vi "Main.vi"() -> ()   [LabVIEW 2025]
uses:
  Resources/States.ctl
  e90cf40e-0b05-4561-bc81-dadeb3f04810.vi
  <vilib>/Utility/file.llb/Write Delimited Spreadsheet (string).vi
  <vilib>/Comparison/Equal/Equal Functor/Equal Functor.lvclass
panel:
  in  "Back PIN":bool
  in  "Change PIN":bool
  in  "New PIN":i32
  in  "Back":bool
  in  "Withdraw":bool
  in  "Withdrawal Amount":dbl
  in  "Log Out":bool
  in  "Withdrawal":bool
  in  "PIN Change":bool
  in  "Balance":bool
  in  "Exit":bool
  in  "Log In":bool
  in  "PIN":i32
  in  "Card Number":i32
  # "ATM MACHINE"
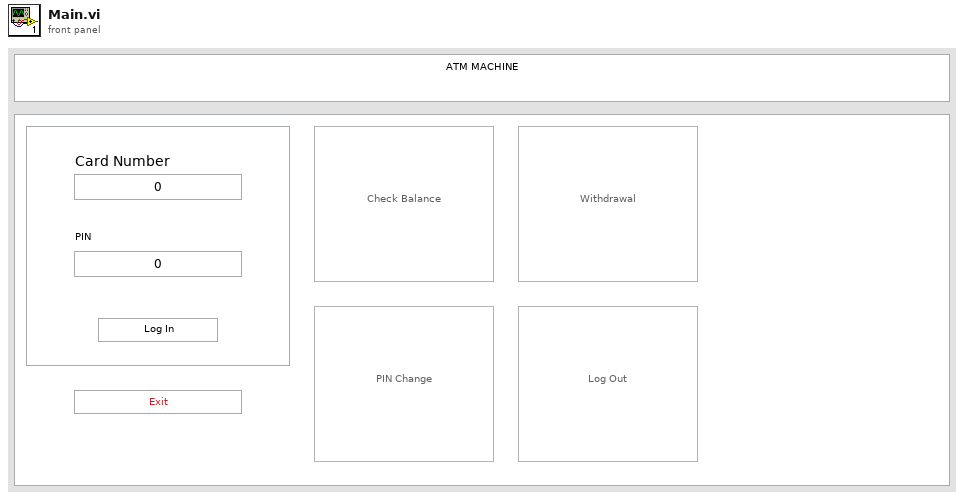
[diagram p1: front panel]
types:
  T1 = cluster{"Card":i32[], "PIN":i32[], "Balance":dbl[], "User Index":i32[]}
  T2 = typedef "States.ctl" = enum16{"Start", "Wait for event", "Log In", "Check Balance", "Withdrawal", "PIN Change", "Money Withdrawal", "Back", "Save File", "New PIN", "Exit Program", "Log Out"}
  T3 = enum16{"open", "replace", "create", "open or create", "replace or create", "replace or create with confirmation"}
  T4 = enum8{"Enabled", "Disabled", "Disabled and Grayed Out"}
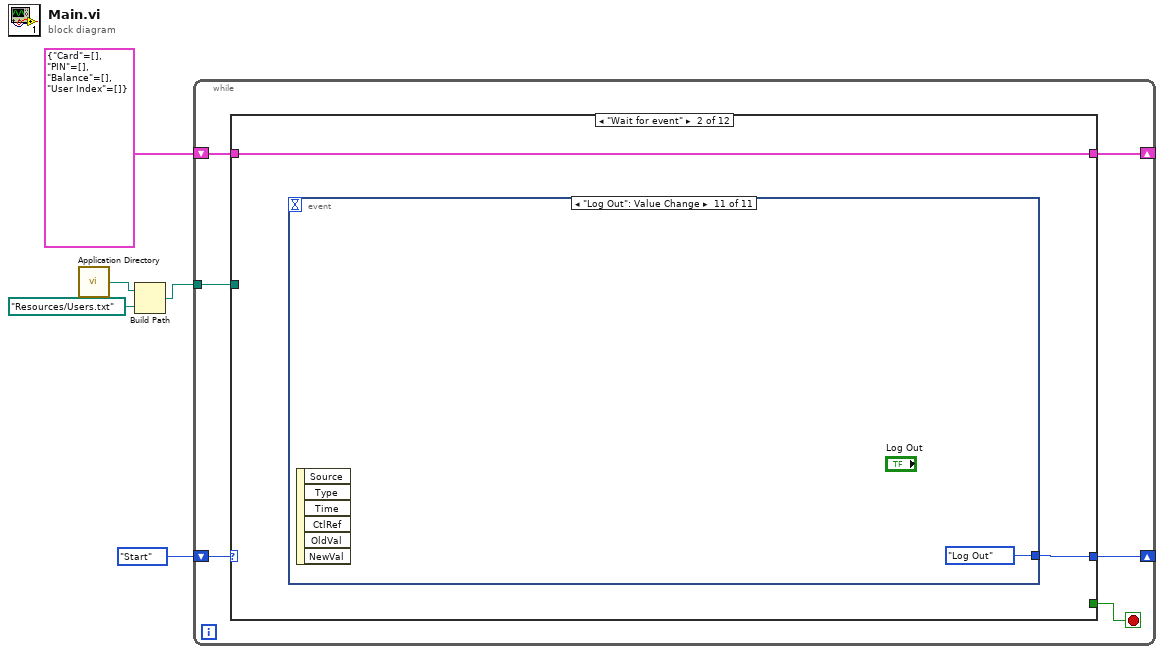
[diagram p0: block diagram]
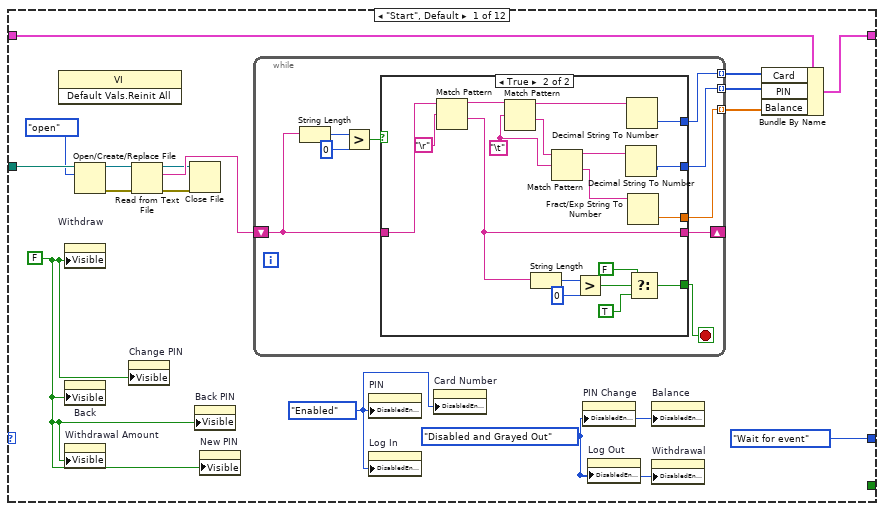
[diagram p2: hidden frame]
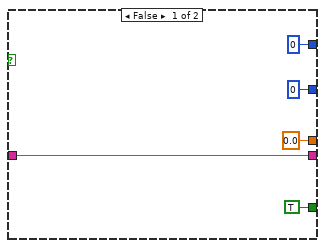
[diagram p3: hidden frame]
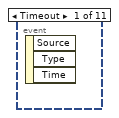
[diagram p4: hidden frame]
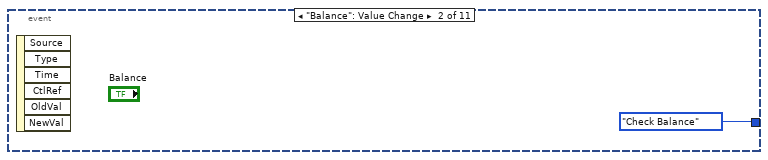
[diagram p5: hidden frame]
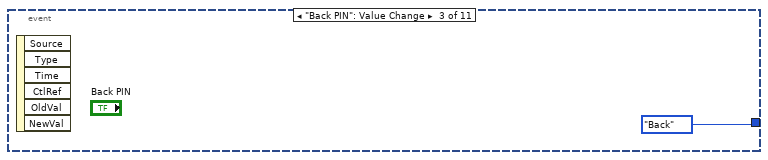
[diagram p6: hidden frame]
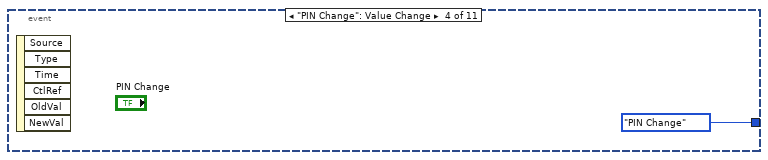
[diagram p7: hidden frame]
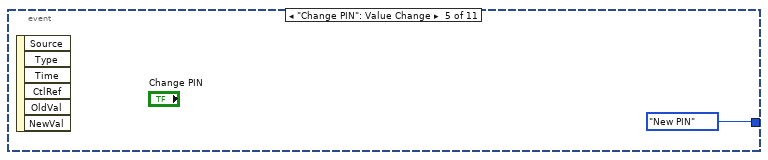
[diagram p8: hidden frame]
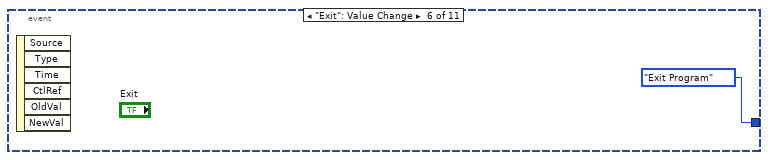
[diagram p9: hidden frame]
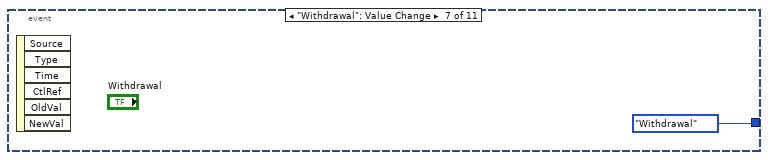
[diagram p10: hidden frame]
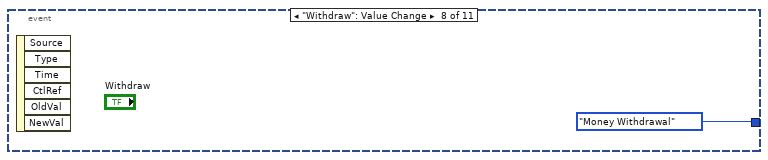
[diagram p11: hidden frame]
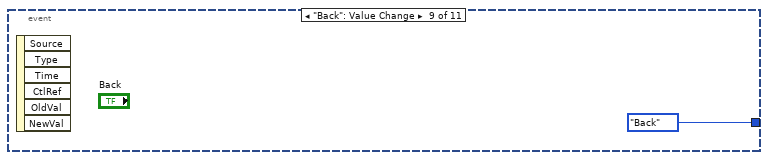
[diagram p12: hidden frame]
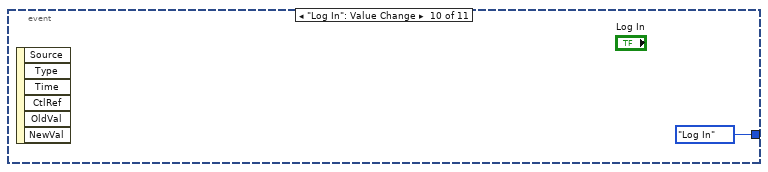
[diagram p13: hidden frame]
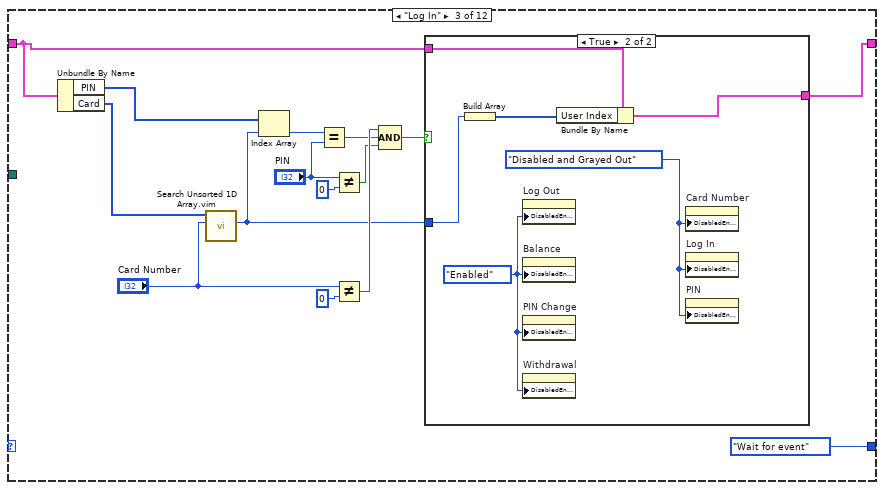
[diagram p14: hidden frame]
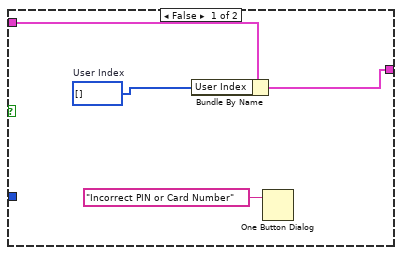
[diagram p15: hidden frame]
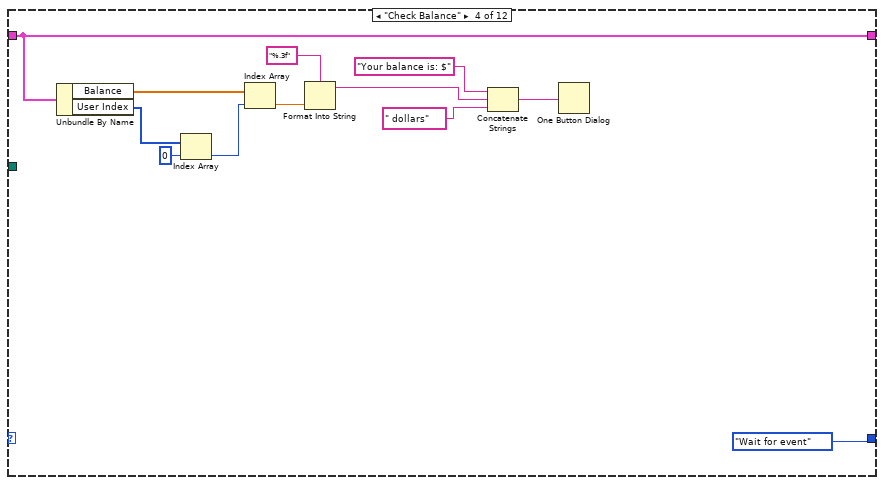
[diagram p16: hidden frame]
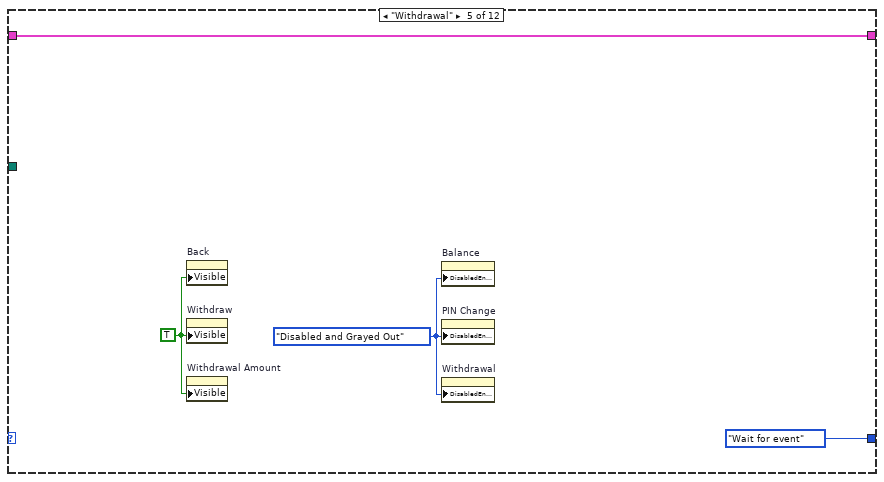
[diagram p17: hidden frame]
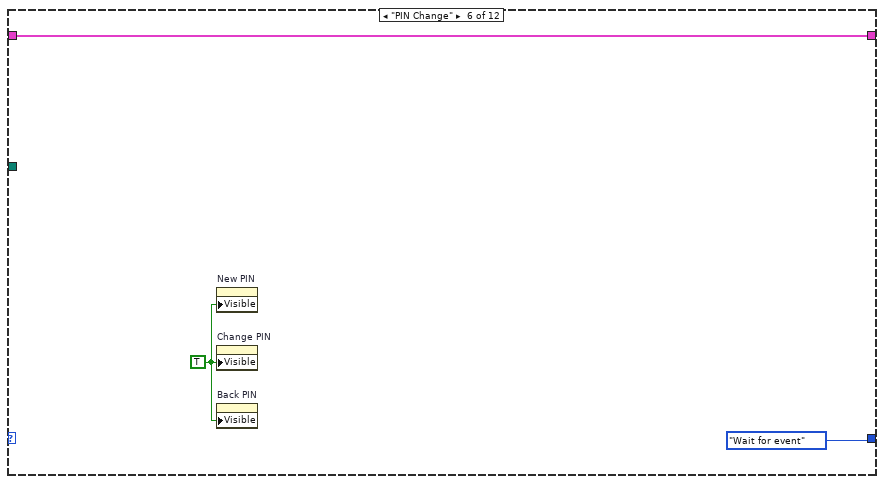
[diagram p18: hidden frame]
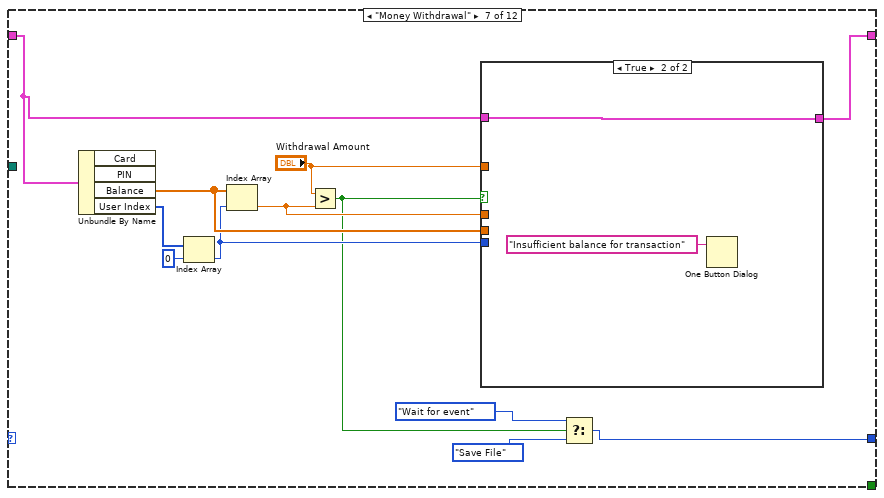
[diagram p19: hidden frame]
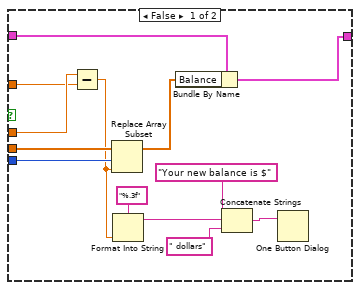
[diagram p20: hidden frame]
diagram:
  n1 = call <vilib>:"Application Directory.vi"() -> ("Application Directory"=w3:path)
  n2 = Build Path(base path=w3, name or relative path=path "Resources/Users.txt") -> (appended path=w1:path)
  n3 = while {
    shift-right: [w10] -> _
    shift-left: States."Start" -> [w11]
    shift-right: [w7] -> _
    shift-left: T1 {"Card"=[], "PIN"=[], "Balance"=[], "User Index"=[]} -> [w8]
    tunnel: w1 -> [w6]
    stop <- w9 stop-if-true
    n4 = case shown="\"Wait for event\"" w11 {
      tunnel: [States."Wait for event" w61 States."Wait for event" States."Wait for event" States."Wait for event" States."Wait for event" w116 States."Wait for event" States."Back" w165 States."Exit Program" States."Start"] -> w10
      tunnel: [_ _ _ _ _ _ _ _ _ _ TRUE _] -> w9
      tunnel: w8 -> [w23 w60 w74 w97 w112 w113 w124 w145 w157 w170 _ _]
      tunnel: [w22 w60 w73 w97 w112 w113 w125 w145 _ w169 _ _] -> w7
      tunnel: w6 -> [w21 _ _ _ _ _ _ _ w148 _ _ _]
      frame "Start", Default {
        w24 = FALSE ("Visible")
        w25 = T4."Disabled and Grayed Out" ("Disabled")
        w26 = T4."Enabled" ("Disabled")
        n5 = invoke class="VI" method="Default Vals.Reinit All"() -> ()  [unwired: 3 in, 3 out]
        n6 = property on="Withdraw" class="Bool"("Visible"=w24) -> ()  [unwired: 2 in, 2 out]
        n7 = property on="Back" class="Bool"("Visible"=w24) -> ()  [unwired: 2 in, 2 out]
        n8 = property on="Withdrawal Amount" class="DigNum (strict)"("Visible"=w24) -> ()  [unwired: 2 in, 2 out]
        n9 = Open/Create/Replace File(file path (use dialog)=w21, operation (0:open)=T3."open") -> (refnum out=w18:refnum<file>, error out=w19:errorcluster)  [unwired: 4 in, 1 out]
        n10 = property on="Change PIN" class="Bool"("Visible"=w24) -> ()  [unwired: 2 in, 2 out]
        n11 = Read from Text File(file (use dialog)=w18, error in=w19) -> (refnum out=w15:refnum<file>, text=w17:string, error out=w16:errorcluster)  [unwired: 2 in, 1 out]
        n12 = Close File(refnum=w15, error in=w16) -> ()  [unwired: 2 out]
        n13 = property on="Back PIN" class="Bool"("Visible"=w24) -> ()  [unwired: 2 in, 2 out]
        n14 = property on="New PIN" class="DigNum (strict)"("Visible"=w24) -> ()  [unwired: 2 in, 2 out]
        n15 = while {
          shift-right: [w36] -> _
          shift-left: w17 -> [w32]
          tunnel: [w30] -> w14 mode=indexing
          tunnel: [w29] -> w13 mode=indexing
          tunnel: [w28] -> w12 mode=indexing
          stop <- w31 stop-if-true
          n16 = String Length(string=w32) -> (length=w35:i32)
          n17 = Greater?(x=w35, y=0) -> (0:w33:bool)
          n18 = case shown="True" w33 {
            tunnel: w32 -> [w41 w59]
            tunnel: [w41 w50] -> w36
            tunnel: [TRUE ("t") w47] -> w31
            tunnel: [0 w45] -> w30
            tunnel: [0 w44] -> w29
            tunnel: [0.0 w43] -> w28
            frame False {
            }
            frame True {
              w42 = "\t"
              n19 = Match Pattern(string=w59, regular expression="\r") -> (before substring=w58:string, after substring=w50:string)  [unwired: 1 in, 2 out]
              n20 = Match Pattern(string=w58, regular expression=w42) -> (before substring=w56:string, after substring=w57:string)  [unwired: 1 in, 2 out]
              n21 = String Length(string=w50) -> (length=w51:i32)
              n22 = Match Pattern(string=w57, regular expression=w42) -> (before substring=w55:string, after substring=w54:string)  [unwired: 1 in, 2 out]
              n23 = Greater?(x=w51, y=0) -> (0:w49:bool)
              n24 = Decimal String To Number(string=w55) -> (number=w44:i32)  [unwired: 2 in, 1 out]
              n25 = Decimal String To Number(string=w56) -> (number=w45:i32)  [unwired: 2 in, 1 out]
              n26 = Fract/Exp String To Number(string=w54) -> (number=w43:dbl)  [unwired: 3 in, 1 out]
              n27 = Select(t=FALSE, s=w49, f=TRUE) -> (s? t:f=w47:bool)
            }
          }
        }
        n28 = property on="PIN" class="DigNum (strict)"("DisabledEnum"=w26) -> ()  [unwired: 2 in, 2 out]
        n29 = property on="Log In" class="Bool"("DisabledEnum"=w26) -> ()  [unwired: 2 in, 2 out]
        n30 = property on="Card Number" class="DigNum (strict)"("DisabledEnum"=w26) -> ()  [unwired: 2 in, 2 out]
        n31 = property on="PIN Change" class="Bool"("DisabledEnum"=w25) -> ()  [unwired: 2 in, 2 out]
        n32 = property on="Log Out" class="Bool"("DisabledEnum"=w25) -> ()  [unwired: 2 in, 2 out]
        n33 = property on="Balance" class="Bool"("DisabledEnum"=w25) -> ()  [unwired: 2 in, 2 out]
        n34 = property on="Withdrawal" class="Bool"("DisabledEnum"=w25) -> ()  [unwired: 2 in, 2 out]
        n35 = Bundle By Name(cluster=w23, "Card"=w14, "PIN"=w13, "Balance"=w12) -> (w22:T1)
      }
      frame "Wait for event" {
        n36 = event shown="[10] \"Log Out\": Value Change" {
          selector: _ -> [_ _ _ _ _ _ _ _ _ _ _]
          dyn-events: _ -> [_ _ _ _ _ _ _ _ _ _ _]
          timeout: _ -> [_ _ _ _ _ _ _ _ _ _ _]
          tunnel: [_ States."Check Balance" States."Back" States."PIN Change" States."New PIN" States."Exit Program" States."Withdrawal" States."Money Withdrawal" States."Back" States."Log In" States."Log Out"] -> w61
          event Timeout {
            n37 = event-data() -> ()  [unwired: 1 in, 3 out]
          }
          event "Balance": Value Change {
            n38 = event-data() -> ()  [unwired: 1 in, 6 out]
          }
          event "Back PIN": Value Change {
            n39 = event-data() -> ()  [unwired: 1 in, 6 out]
          }
          event "PIN Change": Value Change {
            n40 = event-data() -> ()  [unwired: 1 in, 6 out]
          }
          event "Change PIN": Value Change {
            n41 = event-data() -> ()  [unwired: 1 in, 6 out]
          }
          event "Exit": Value Change {
            n42 = event-data() -> ()  [unwired: 1 in, 6 out]
          }
          event "Withdrawal": Value Change {
            n43 = event-data() -> ()  [unwired: 1 in, 6 out]
          }
          event "Withdraw": Value Change {
            n44 = event-data() -> ()  [unwired: 1 in, 6 out]
          }
          event "Back": Value Change {
            n45 = event-data() -> ()  [unwired: 1 in, 6 out]
          }
          event "Log In": Value Change {
            n46 = event-data() -> ()  [unwired: 1 in, 6 out]
          }
          event "Log Out": Value Change {
            n47 = event-data() -> ()  [unwired: 1 in, 6 out]
          }
        }
      }
      frame "Log In" {
        n48 = Unbundle By Name(w74) -> ("PIN"=w76:i32[], "Card"=w75:i32[])
        n49 = call "Search Unsorted 1D Array.vim"("element"="Card Number", "unsorted 1D array"=w75) -> ("index of element"=w72:i32)  [unwired: 9 in]
        n50 = Index Array(array=w76, index=w72) -> (element=w86:i32)
        n51 = Equal?(x=w86, y="PIN") -> (x = y?=w80:bool)
        n52 = Not Equal?(x="PIN", y=0) -> (x != y?=w79:bool)
        n53 = Not Equal?(x="Card Number", y=0) -> (x != y?=w81:bool)
        n54 = Compound Arithmetic op=AND(w81, w80, w79) -> (w78:bool)
        n55 = case shown="True" w78 {
          tunnel: w74 -> [w89 w94]
          tunnel: [w88 w93] -> w73
          tunnel: w72 -> [_ w92]
          frame False {
            w87 = i32[] []  # User Index
            n56 = Bundle By Name(cluster=w89, "User Index"=w87) -> (w88:T1)
            n57 = One Button Dialog(message="Incorrect PIN or Card Number") -> ()  [unwired: 1 in, 1 out]
          }
          frame True {
            w95 = T4."Disabled and Grayed Out" ("Disabled")
            w96 = T4."Enabled" ("Disabled")
            n58 = Build Array(w92) -> (w91:i32[])
            n59 = property on="Log Out" class="Bool"("DisabledEnum"=w96) -> ()  [unwired: 2 in, 2 out]
            n60 = property on="Balance" class="Bool"("DisabledEnum"=w96) -> ()  [unwired: 2 in, 2 out]
            n61 = property on="PIN Change" class="Bool"("DisabledEnum"=w96) -> ()  [unwired: 2 in, 2 out]
            n62 = property on="Withdrawal" class="Bool"("DisabledEnum"=w96) -> ()  [unwired: 2 in, 2 out]
            n63 = Bundle By Name(cluster=w94, "User Index"=w91) -> (w93:T1)
            n64 = property on="Card Number" class="DigNum (strict)"("DisabledEnum"=w95) -> ()  [unwired: 2 in, 2 out]
            n65 = property on="Log In" class="Bool"("DisabledEnum"=w95) -> ()  [unwired: 2 in, 2 out]
            n66 = property on="PIN" class="DigNum (strict)"("DisabledEnum"=w95) -> ()  [unwired: 2 in, 2 out]
          }
        }
      }
      frame "Check Balance" {
        n67 = Unbundle By Name(w97) -> ("Balance"=w108:dbl[], "User Index"=w107:i32[])
        n68 = Index Array(array=w107, index=0) -> (element=w105:i32)
        n69 = Index Array(array=w108, index=w105) -> (element=w104:dbl)
        n70 = Format Into String(format string="%.3f", w104) -> (resulting string=w101:string)  [unwired: 2 in, 1 out]
        n71 = Concatenate Strings("Your balance is: $", w101, " dollars") -> (w99:string)
        n72 = One Button Dialog(message=w99) -> ()  [unwired: 1 in, 1 out]
      }
      frame "Withdrawal" {
        w109 = T4."Disabled and Grayed Out" ("Disabled")
        w111 = TRUE ("Visible")
        n73 = property on="Back" class="Bool"("Visible"=w111) -> ()  [unwired: 2 in, 2 out]
        n74 = property on="Withdraw" class="Bool"("Visible"=w111) -> ()  [unwired: 2 in, 2 out]
        n75 = property on="Withdrawal Amount" class="DigNum (strict)"("Visible"=w111) -> ()  [unwired: 2 in, 2 out]
        n76 = property on="Balance" class="Bool"("DisabledEnum"=w109) -> ()  [unwired: 2 in, 2 out]
        n77 = property on="PIN Change" class="Bool"("DisabledEnum"=w109) -> ()  [unwired: 2 in, 2 out]
        n78 = property on="Withdrawal" class="Bool"("DisabledEnum"=w109) -> ()  [unwired: 2 in, 2 out]
      }
      frame "PIN Change" {
        w115 = TRUE ("Visible")
        n79 = property on="New PIN" class="DigNum (strict)"("Visible"=w115) -> ()  [unwired: 2 in, 2 out]
        n80 = property on="Change PIN" class="Bool"("Visible"=w115) -> ()  [unwired: 2 in, 2 out]
        n81 = property on="Back PIN" class="Bool"("Visible"=w115) -> ()  [unwired: 2 in, 2 out]
      }
      frame "Money Withdrawal" {
        n82 = Unbundle By Name(w124) -> ("Balance"=w121:dbl[], "User Index"=w127:i32[])  [unwired: 2 out]
        n83 = Index Array(array=w127, index=0) -> (element=w120:i32)
        n84 = Index Array(array=w121, index=w120) -> (element=w123:dbl)
        n85 = Greater?(x="Withdrawal Amount", y=w123) -> (0:w119:bool)
        n86 = case shown="True" w119 {
          tunnel: [w135 w142] -> w125
          tunnel: w124 -> [w136 w142]
          tunnel: w123 -> [w140 _]
          tunnel: "Withdrawal Amount" -> [w139 _]
          tunnel: w121 -> [w138 _]
          tunnel: w120 -> [w137 _]
          frame False {
            n87 = Subtract(x=w140, y=w139) -> (x-y=w133:dbl)
            n88 = Replace Array Subset(array=w138, new element=w133, index=w137) -> (w134:dbl[])
            n89 = Format Into String(format string="%.3f", w133) -> (resulting string=w130:string)  [unwired: 2 in, 1 out]
            n90 = Bundle By Name(cluster=w136, "Balance"=w134) -> (w135:T1)
            n91 = Concatenate Strings("Your new balance is $" ("string"), w130, " dollars" ("string")) -> (w128:string)
            n92 = One Button Dialog(message=w128) -> ()  [unwired: 1 in, 1 out]
          }
          frame True {
            n93 = One Button Dialog(message="Insufficient balance for transaction") -> ()  [unwired: 1 in, 1 out]
          }
        }
        n94 = Select(t=States."Wait for event", s=w119, f=States."Save File") -> (s? t:f=w116:T2)
      }
      frame "Back" {
        w144 = T4."Enabled" ("Disabled")
        w143 = FALSE ("Visible")
        n95 = property on="Withdraw" class="Bool"("Visible"=w143) -> ()  [unwired: 2 in, 2 out]
        n96 = property on="Back" class="Bool"("Visible"=w143) -> ()  [unwired: 2 in, 2 out]
        n97 = property on="New PIN" class="DigNum (strict)"("Visible"=w143) -> ()  [unwired: 2 in, 2 out]
        n98 = property on="Back PIN" class="Bool"("Visible"=w143) -> ()  [unwired: 2 in, 2 out]
        n99 = property on="Change PIN" class="Bool"("Visible"=w143) -> ()  [unwired: 2 in, 2 out]
        n100 = property on="Withdrawal Amount" class="DigNum (strict)"("Visible"=w143) -> ()  [unwired: 2 in, 2 out]
        n101 = property on="PIN Change" class="Bool"("DisabledEnum"=w144) -> ()  [unwired: 2 in, 2 out]
        n102 = property on="Balance" class="Bool"("DisabledEnum"=w144) -> ()  [unwired: 2 in, 2 out]
        n103 = property on="Withdrawal" class="Bool"("DisabledEnum"=w144) -> ()  [unwired: 2 in, 2 out]
      }
      frame "Save File" {
        n104 = Unbundle By Name(w157) -> ("Card"=w156:i32[], "PIN"=w155:i32[], "Balance"=w154:dbl[])
        n105 = for {
          tunnel: w156 -> [w164] mode=indexing
          tunnel: w155 -> [w163] mode=indexing
          tunnel: w154 -> [w162] mode=indexing
          tunnel: [w160] -> w153 mode=indexing
          tunnel: [w159] -> w152 mode=indexing
          tunnel: [w158] -> w151 mode=indexing
          n106 = Format Into String(w163) -> (resulting string=w159:string)  [unwired: 3 in, 1 out]
          n107 = Format Into String(w164) -> (resulting string=w160:string)  [unwired: 3 in, 1 out]
          n108 = Format Into String(format string="%.3f", w162) -> (resulting string=w158:string)  [unwired: 2 in, 1 out]
        }
        n109 = Build Array(w153, w152, w151) -> (w150:string[][])
        n110 = Transpose 2D Array(2D array=w150) -> (transposed array=w149:string[][])
        n111 = call-poly <vilib>:"Write Delimited Spreadsheet.vi"("file path (dialog if empty)"=w148, "2D data"=w149) -> ()  [unwired: 12 in, 2 out]
      }
      frame "New PIN" {
        n112 = Unbundle By Name(w170) -> ("PIN"=w176:i32[], "User Index"=w178:i32[])
        n113 = Index Array(array=w178, index=0) -> (element=w171:i32)
        n114 = Format Into String("New PIN") -> (resulting string=w174:string)  [unwired: 3 in, 1 out]
        n115 = String Length(string=w174) -> (length=w173:i32)
        n116 = Not Equal?(x=w173, y=4) -> (x != y?=w168:bool)
        n117 = case shown="True" w168 {
          tunnel: w176 -> [w187 _]
          tunnel: "New PIN" -> [w182 _]
          tunnel: w171 -> [w183 _]
          tunnel: w170 -> [w186 w188]
          tunnel: [w184 w188] -> w169
          frame False {
            n118 = Replace Array Subset(array=w187, new element=w182, index=w183) -> (w185:i32[])
            n119 = Format Into String(w182) -> (resulting string=w181:string)  [unwired: 3 in, 1 out]
            n120 = Bundle By Name(cluster=w186, "PIN"=w185) -> (w184:T1)
            n121 = Concatenate Strings("Your new PIN is " ("string"), w181) -> (w179:string)
            n122 = One Button Dialog(message=w179) -> ()  [unwired: 1 in, 1 out]
          }
          frame True {
            n123 = One Button Dialog(message="The PIN must be four digits long") -> ()  [unwired: 1 in, 1 out]
          }
        }
        n124 = Select(t=States."Wait for event", s=w168, f=States."Save File") -> (s? t:f=w165:T2)
      }
      frame "Exit Program" {
      }
      frame "Log Out" {
      }
    }
  }
